vi "Disconnect.vi"(8 "error in":errorcluster, 11 "4081 in":refnum<class "4081.lvclass">) -> (0 "error out":errorcluster, 3 "4081 out":refnum<class "4081.lvclass">)   [LabVIEW 2019, in "4081.lvlib" / "4081.lvclass"]
uses:
  Library/4081.lvclass
  Library/4081.lvclass/4081.ctl
  builds/Instruments/Multimeter.lvlibp/Library/Multimeter.lvclass
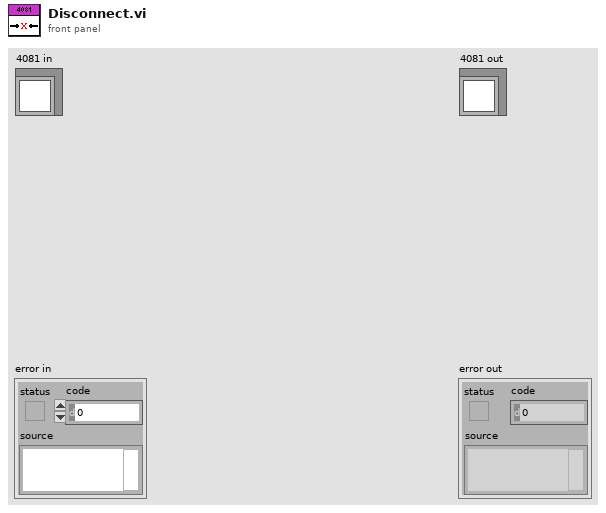
[diagram p1: front panel]
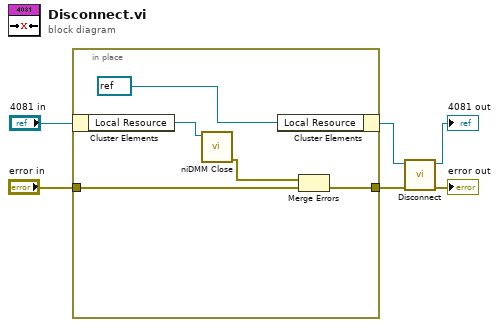
[diagram p0: block diagram]
diagram:
  n1 = in-place {
    in-place-border: "error in" -> [w8]
    in-place-border: [w7] -> w1
    n2 = in-place-cluster #1("4081 in") -> ("Local Resource"=w11:refnum<k15>)
    n3 = call <instrlib>:"niDMM Close.vi"("instrument handle"=w11) -> ("error out"=w9:errorcluster)  [unwired: 10 in]
    n4 = in-place-cluster #1("Local Resource"=refnum<k15> refnum) -> (w2:refnum<class "4081.lvclass">)
    n5 = Merge Errors(w9, w8) -> (w7:errorcluster)
  }
  n6 = call-parent "Disconnect.vi"("error in"=w1, "Multimeter in"=w2) -> ("error out"=→"error out":errorcluster, "Multimeter out"=→"4081 out":refnum<class "4081.lvclass">)  [unwired: 8 in]
